vi "EventsMessage.vi"() -> ()   [LabVIEW 2017]
uses:
  EventMessage.ctl
panel:
  in  "EventsMessage":T1
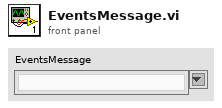
[diagram p1: front panel]
types:
  T1 = typedef "EventMessage.ctl" = string
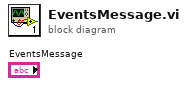
[diagram p0: block diagram]
diagram:
